vi "ByRef Parallel Unbundle.vi"   [LabVIEW 2018]
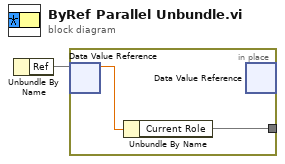
[diagram p0: block diagram]
diagram:
  n1 = Unbundle By Name() -> ("Ref"=w1)  [unwired: 1 in]
  n2 = in-place {
    in-place-border: [w2] -> _
    n3 = in-place-dvr #1(w1) -> (w3:dbl)  [unwired: 1 out]
    n4 = Unbundle By Name(w3) -> ("Current Role"=w2)
    n5 = in-place-dvr #1() -> ()  [unwired: 1 in, 2 out]
  }
